vi "01 HEWH Testing.vi"() -> ()   [LabVIEW 2009]
uses:
  EquipReferences.ctl
panel:
  out "Temp,Humidity Chart":T1(graph)
  in  "Humidity":dbl[](array[numeric])=[50.0, 50.0, 50.0, 50.0]
  in  "Ambient Temp":dbl[](array[numeric])=[58.0, 58.0, 58.0, 58.0]
  out "Elapsed Time":dbl format="%<%H:%M:%S>t"
  out "Stop":bool=TRUE
  in  "H2O Degrees":dbl[](array[numeric])=[58.0, 58.0, 58.0, 58.0]
  in  "Flow Rate":dbl[](array[numeric])=[3.0, 3.0, 3.0, 3.0]
  out "Current Test":i32
  in  "Semiphore":T2
  in  "Test Array":T3(array[ring])=[enum."Mini Heat Up", enum."Mini Heat Up", enum."Mini Heat Up", enum."Mini Heat Up"]
  in  "Equipment":T4={"COM Port"="COM5", "MW100"="MW100", "AG34970"="A-34972A", "Chamber"="Tenney35"}
  out "Error Out":errorcluster
  in  "Error In":errorcluster
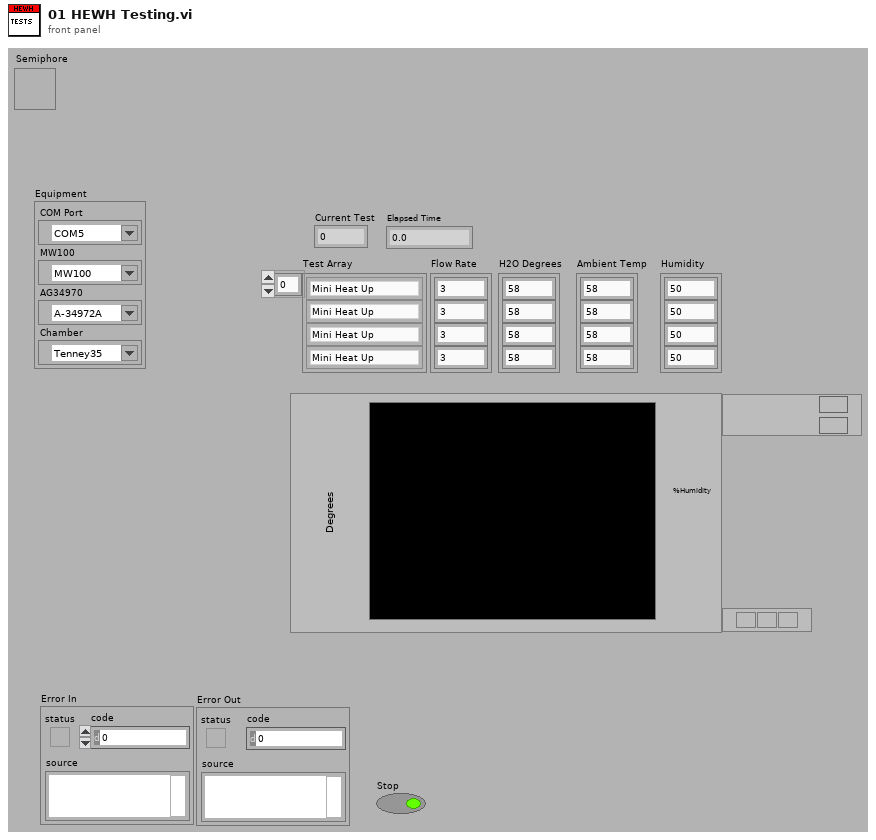
[diagram p1: front panel]
types:
  T1 = cluster{"[0]":dbl, "[1]":dbl, "[2]":dbl, "[3]":dbl, "[4]":dbl, "[5]":dbl}
  T2 = typedef "Semaphore RefNum" = refnum<k1>
  T3 = enum16{"Heat Up Test", "24 Hour Test", "First Hour Delivery", "Mini Heat Up"}[]
  T4 = typedef "EquipReferences.ctl" = cluster{"COM Port":refnum<visa-resource-name>, "MW100":refnum<visa-resource-name>, "AG34970":refnum<visa-resource-name>, "Chamber":refnum<visa-resource-name>}
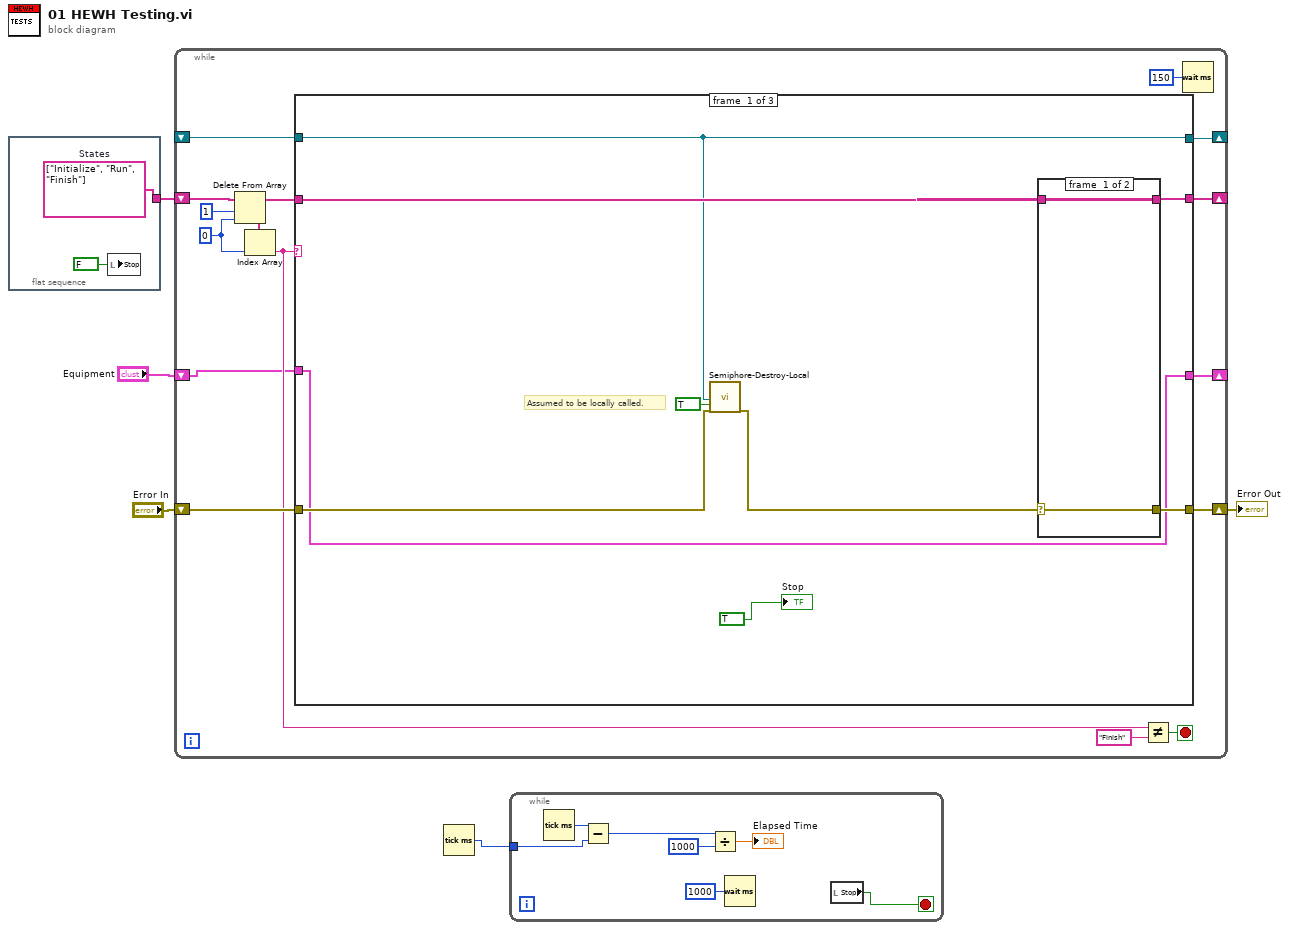
[diagram p0: block diagram]
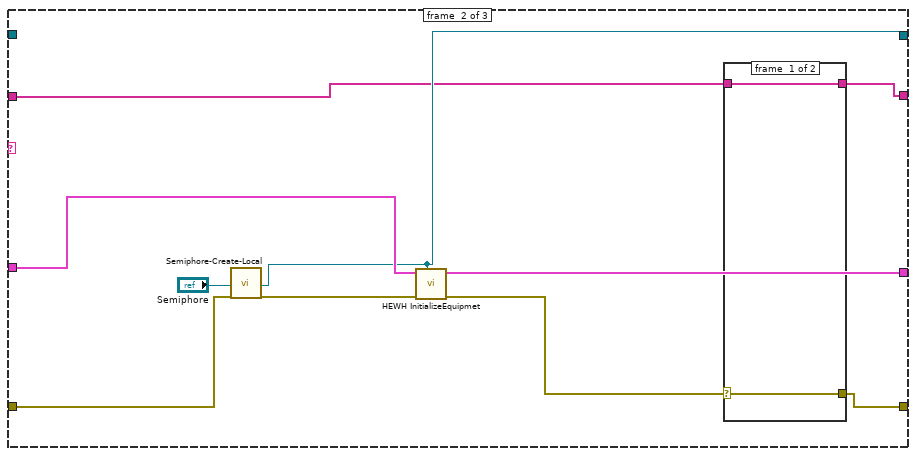
[diagram p3: hidden frame]
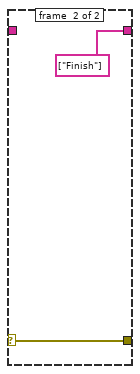
[diagram p4: hidden frame]
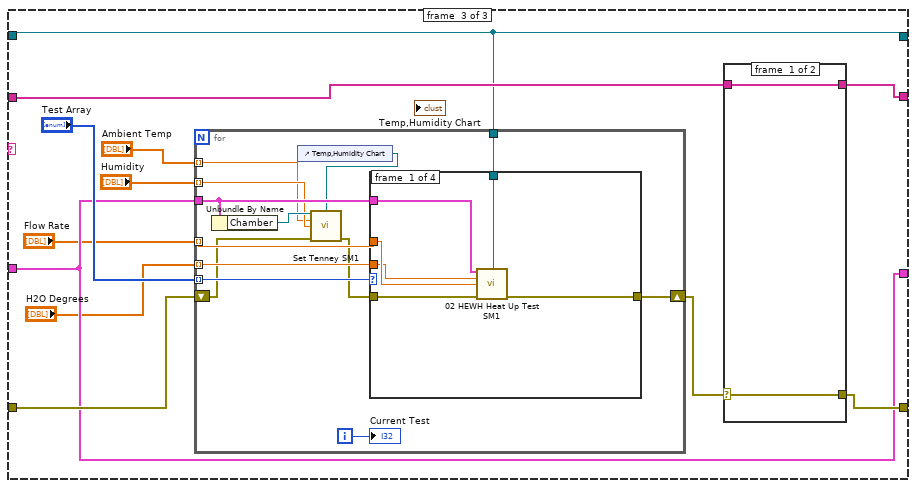
[diagram p5: hidden frame]
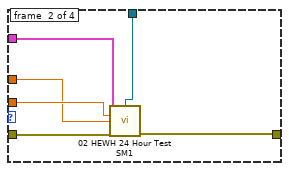
[diagram p6: hidden frame]
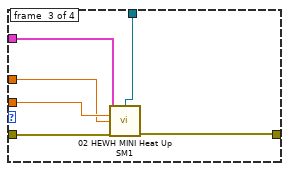
[diagram p7: hidden frame]
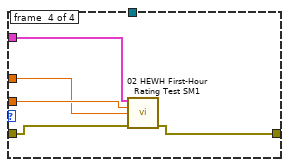
[diagram p8: hidden frame]
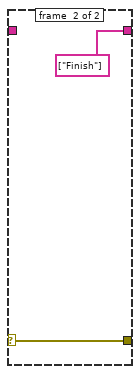
[diagram p9: hidden frame]
diagram:
  n1 = flat-sequence {
    tunnel: [w7] -> w5
    frame #0 {
      w7 = string[] ["Initialize", "Run", "Finish"]  # States
      n2 = local write "Stop"(FALSE ("Stop")) -> ()
    }
  }
  n3 = while {
    shift-right: [w19] -> _
    shift-left: w5 -> [w23]
    shift-right: [w16] -> w3
    shift-left: "Error In" -> [w15]
    shift-right: [w11] -> _
    shift-left: "Equipment" -> [w8]
    shift-right: [w10] -> _
    shift-left: _ -> [w9]
    stop <- w14 stop-if-true
    w20 = 0 ("index")
    n4 = Delete From Array(array=w23, length=1, index=w20) -> (deleted portion=w21:string[], array with subset deleted=w18:string[])
    n5 = Index Array(array=w21, index=w20) -> (element=w13:string)
    n6 = case shown="\"Run\"" w13 {
      tunnel: [w32 w39 w61] -> w19
      tunnel: w18 -> [w31 w40 w62]
      tunnel: [w30 w37 w60] -> w16
      tunnel: w15 -> [w29 w42 w58]
      tunnel: w8 -> [w25 w44 w56]
      tunnel: [w25 w43 w56] -> w11
      tunnel: [w27 w41 w55] -> w10
      tunnel: w9 -> [w27 _ w55]
      frame #0 {
        # "Assumed to be locally called."
        n7 = call "Semiphore-Destroy-Local.vi"("Semiphore"=w27, "Local?"=TRUE, "error in (no error)"=w29) -> ("error out"=w28:errorcluster)  [unwired: 16 in]
        n8 = case shown="Error" w28 {
          selector: w28 -> [w33 w35]
          tunnel: [w34 w36] -> w32
          tunnel: w31 -> [w34 w36]
          tunnel: [w33 w35] -> w30
          frame #0 {
          }
          frame #1 {
          }
        }
        "Stop" <- TRUE
      }
      frame #1 {
        n9 = call "Semiphore-Create-Local.vi"("Semiphore"="Semiphore", "error in (no error)"=w42) -> ("semaphore"=w41:T2, "error out"=w45:errorcluster)  [unwired: 15 in, 1 out]
        n10 = call "HEWH InitializeEquipmet.vi"("Semiphore"=w41, "Error In"=w45, "Equipment"=w44) -> ("Error Out"=w38:errorcluster, "Equipment Out"=w43:T4)  [unwired: 6 in, 1 out]
        n11 = case shown="Error" w38 {
          selector: w38 -> [w47 w50]
          tunnel: [w48 string[] ["Finish"] ("States")] -> w39
          tunnel: w40 -> [w48 _]
          tunnel: [w47 w50] -> w37
          frame #0 {
          }
          frame #1 {
          }
        }
      }
      frame #2 {
        n12 = for {
          tunnel: "Test Array" -> [w75] mode=indexing
          shift-right: [w74] -> w57
          shift-left: w58 -> [w69]
          tunnel: w56 -> [w67]
          tunnel: w55 -> [w73]
          tunnel: "Flow Rate" -> [w72] mode=indexing
          tunnel: "H2O Degrees" -> [w71] mode=indexing
          tunnel: "Humidity" -> [w65] mode=indexing
          tunnel: "Ambient Temp" -> [w64] mode=indexing
          i -> [w70]
          n13 = Unbundle By Name(w67) -> ("Chamber"=w66:refnum<visa-resource-name>)
          n14 = control-ref of="Temp,Humidity Chart"() -> (w63:refnum<vi>)
          n15 = call "Set Tenney SM1.vi"("Interface\nType"=w66, "Temp,Humidity ChartOut"=w63, "Temp Set Point"=w64, "Humidity Set Point"=w65, "Error In"=w69) -> ("Error Out"=w68:errorcluster)  [unwired: 8 in, 2 out]
          n16 = case shown="\"Heat Up Test\", Default" w75 {
            tunnel: w68 -> [w81 w87 w93 w98]
            tunnel: [w80 w86 w92 w97] -> w74
            tunnel: w67 -> [w79 w82 w88 w96]
            tunnel: w73 -> [w78 w85 w91 _]
            tunnel: w72 -> [w77 w83 w89 w94]
            tunnel: w71 -> [w76 w84 w90 w95]
            frame #0 {
              n17 = call "02 HEWH Heat Up Test SM1.vi"("Equipment"=w79, "Semiphore"=w78, "Degree Setting"=w76, "Flow rate setting"=w77, "Error In"=w81) -> ("Error Out"=w80:errorcluster)  [unwired: 10 in]
            }
            frame #1 {
              n18 = call "02 HEWH 24 Hour Test SM1.vi"("Equipment"=w82, "Semiphore"=w85, "Degree Setting"=w84, "Flow rate setting"=w83, "Error In"=w87) -> ("Error Out"=w86:errorcluster)  [unwired: 10 in]
            }
            frame #2 {
              n19 = call "02 HEWH MINI Heat Up SM1.vi"("Equipment"=w88, "Semiphore"=w91, "Degree Setting"=w90, "Flow rate setting"=w89, "Error In"=w93) -> ("Error Out"=w92:errorcluster)  [unwired: 10 in]
            }
            frame #3 {
              n20 = call "02 HEWH First-Hour Rating Test SM1.vi"("Equipment"=w96, "Degree Setting"=w95, "Flow rate setting"=w94, "Error In"=w98) -> ("Error Out"=w97:errorcluster)  [unwired: 11 in]
            }
          }
          "Current Test" <- w70
        }
        n21 = case shown="Error" w57 {
          selector: w57 -> [w99 w102]
          tunnel: [w100 string[] ["Finish"] ("States")] -> w61
          tunnel: w62 -> [w100 _]
          tunnel: [w99 w102] -> w60
          frame #0 {
          }
          frame #1 {
          }
        }
      }
    }
    n22 = Not Equal?(x=w13, y="Finish") -> (x != y?=w14:bool)
    n23 = Wait (ms)(milliseconds to wait=u32 150) -> ()  [unwired: 1 out]
  }
  "Error Out" <- w3
  n24 = Tick Count (ms)() -> (millisecond timer value=w1:u32)
  n25 = while {
    tunnel: w1 -> [w105]
    stop <- w109 stop-if-true
    n26 = Tick Count (ms)() -> (millisecond timer value=w106:u32)
    n27 = Subtract(x=w106, y=w105) -> (x-y=w104:u32)
    n28 = Divide(x=w104, y=u32 1000) -> (x/y=→"Elapsed Time":dbl)
    n29 = Wait (ms)(milliseconds to wait=u32 1000) -> ()  [unwired: 1 out]
    n30 = local read "Stop"() -> (w109:bool)
  }
